vi "Day 8-2.vi"() -> ()   [LabVIEW 2019, in "Day 8.lvlib"]
uses:
  Day 8.lvlib
panel:
  out "Array 2":string[](array[string])=["4071", "6468", "3280", "8950", "2870", "3397", "3219", "7938", "9511", "6798", "2769", "3672", "6734", "0784", "4865", "7172", "1948", "3386", "6394", "6035", "6388", "4268", "5479", "3876", "9799", "2603", "7009", "2937", "8421", "2344", "6241", "3548", "9654", "4281", "2324", "3134", "1290", "2001", "6508", "3774", "2051", "8563", "6678", "9605", "9989", "6560", "5968", "0362", "3584", "8891", "4895", "8699", "2381", "9222", "1822", "5228", "1804", "0780", "9704", "9642", "2495", "4224", "0930", "3262", "3312", "9354", "9007", "1129", "1990", "5179", "8301", "5799", "8661", "6508", "4845", "6988", "8258", "9544", "0971", "3310", "8569", "1471", "9270", "1287", "7671", "0011", "0695", "1654", "2588", "9727", "1006", "9039", "2552", "5249", "3745", "3553", "3225", "8583", "4118", "3505", "6532", "5649", "3087", "8540", "7804", "6876", "7351", "1683", "8021", "2539", "2269", "0445", "7004", "5965", "3168", "3507", "5671", "3405", "6663", "3932", "1907", "1881", "6367", "0693", "1303", "7941", "1632", "0300", "4682", "0436", "9530", "0970", "2408", "0964", "3910", "9995", "1594", "0618", "7537", "2638", "4820", "6626", "2007", "8972", "4462", "0209", "4073", "9919", "4147", "2885", "6588", "3629", "1539", "0686", "7248", "1846", "0806", "9160", "6565", "9606", "5448", "1654", "8728", "7302", "9365", "5351", "1478", "9649", "3370", "6871", "0242", "3636", "4933", "6608", "5974", "7251", "2822", "5889", "2763", "9681", "2230", "1352", "2526", "3487", "4732", "5051", "0132", "6767", "1347", "2326", "2292", "0408", "2225", "6385", "0328", "2206", "5424", "2763", "3506", "8859"]
  out "Array":i32[](array[numeric])=[4071, 6468, 3280, 8950, 2870, 3397, 3219, 7938, 9511, 6798, 2769, 3672, 6734, 784, 4865, 7172, 1948, 3386, 6394, 6035, 6388, 4268, 5479, 3876, 9799, 2603, 7009, 2937, 8421, 2344, 6241, 3548, 9654, 4281, 2324, 3134, 1290, 2001, 6508, 3774, 2051, 8563, 6678, 9605, 9989, 6560, 5968, 362, 3584, 8891, 4895, 8699, 2381, 9222, 1822, 5228, 1804, 780, 9704, 9642, 2495, 4224, 930, 3262, 3312, 9354, 9007, 1129, 1990, 5179, 8301, 5799, 8661, 6508, 4845, 6988, 8258, 9544, 971, 3310, 8569, 1471, 9270, 1287, 7671, 11, 695, 1654, 2588, 9727, 1006, 9039, 2552, 5249, 3745, 3553, 3225, 8583, 4118, 3505, 6532, 5649, 3087, 8540, 7804, 6876, 7351, 1683, 8021, 2539, 2269, 445, 7004, 5965, 3168, 3507, 5671, 3405, 6663, 3932, 1907, 1881, 6367, 693, 1303, 7941, 1632, 300, 4682, 436, 9530, 970, 2408, 964, 3910, 9995, 1594, 618, 7537, 2638, 4820, 6626, 2007, 8972, 4462, 209, 4073, 9919, 4147, 2885, 6588, 3629, 1539, 686, 7248, 1846, 806, 9160, 6565, 9606, 5448, 1654, 8728, 7302, 9365, 5351, 1478, 9649, 3370, 6871, 242, 3636, 4933, 6608, 5974, 7251, 2822, 5889, 2763, 9681, 2230, 1352, 2526, 3487, 4732, 5051, 132, 6767, 1347, 2326, 2292, 408, 2225, 6385, 328, 2206, 5424, 2763, 3506, 8859]
  out "Resolt":i32=940724
  out "array":string[][](array[string])=[["ecgabfd gfbe dgbeaf aeg gfbda eg bgdcaf efgdca abced eadgb", " begf decgfa aeg eg"], ["ebfg bfgdea gaf gf baedgc dafec cfdabg ecfabgd fdgea dbaeg", " gaedbc egbf dbgcea dagfebc"], ["cfadeg ca bacg dfabe dgcbf dbegafc dac afbdgc gcbedf bfcda", " fbdac adbef bgcdfae dcagfe"], ["eag cdgfae cbdge ae fcgad eabdfg ecaf gefbadc dgafcb degca", " dacbefg fcdage agdcf fedagb"], ["dga edac gdfbea bgdfec da cfbga dbgec cadgb bdgace dcbfage", " acgfb gaecbfd dag gedfab"], ["cefb fb abcgefd fagbde fcbgae faecg cbadg cbfga bfa agcdef", " gbacf agbfc bgcaef baf"], ["ebdacf cbgfae cgdebaf afdcb gabdc df cdf eafd ecabf begdfc", " cbdaf gdabc fd cbefda"], ["ge daebc fcagb fdebac gaed ecabg egc gacedb cbdfeg adcfbeg", " gec gebdca ebagc adbgcfe"], ["bgfade gcefbd eafgd fcae cadgf gcf dgcba cfdega cagbdfe cf", " cdgeaf agfed cf cf"], ["abfge ebac acfegbd bc fcged gbfec cfgbad fecabg agbfde fcb", " aefgdb cfb egbfca cbfaedg"], ["dfcbag gda dcafe gcdeb ag ecgdaf edagc bcdaef gcbadfe gaef", " gbced dga cbadef fgecda"], ["cagb adgceb cdb cfgeda egfbd abcefd decag bc cgebd bgedfca", " cegbd dfegac dbc befdg"], ["cbfe bgefdc ceabdfg cf dbgaef gdfbac edcga gcfed dfc fbedg", " fgbaed fcd fcegd becf"], ["degabf bfg bcgaf gdacf dbfc gecfda gcaeb fagedbc adfgbc bf", " egbdfa gbf adfbceg dcfb"], ["dbfae dfbc ecadg cb cbdea fcebag fgadbec gadebf bec ceabfd", " dbfc bgfcead agbedf fdabe"], ["dafcge ecafbg cegaf egdac abegd cd debfca edc cgfd bfdeagc", " dec dc ecd dbgae"], ["fgabce bfa acbfegd fcegda bfgd acgfd bcaed bfcda bf cbagdf", " bf bafgcd bfdg dgbacfe"], ["fgea gad fcbgaed gdebc afdeb fagcbd cbfeda ag egfdba degab", " dgeab badge eacfbdg fdceba"], ["fabdce cagdb gcb bcefag degba dfagbc dgcf dcfab egfcabd cg", " befcda dbagc cbdgfa gcdf"], ["be fgaced fdeag badegf fdbea ebdg bea agfbec ebgadcf bcfad", " acdfge agbfce debaf dgafe"], ["cdfbeg bg fegca gdefac cadbf eadbcgf cgb egba gcfbea cagfb", " gfaced agfcb cbdfaeg cgfdabe"], ["fadcebg cgda ebfag adebc fcebdg fadbce gd begcda bdg gedba", " dcga fbage dcabef fcebadg"], ["bfcga adfbgc fbcdage gfedac ab gcfbe cgafd efabgd gab bdca", " gcafd cdba gba dfabgc"], ["bdfae gfa cdgabe egfba fg gfeadc acegb fgcb fbecgad ecafgb", " bgeaf agfecbd fga agdceb"], ["dgab ebfad cdefgb gbefd fab cefabg fegcbda aedcf ba ebadgf", " defbag afb gbfead dbefag"], ["cfabed ecabf cgafdeb bfc fecbgd dcab cb bfeda eagfc adfgeb", " fgcae dfbega ebcdfg fabec"], ["eb cbgaef eagcfbd caebd gaedbc badfc abe degac dgeb cgdeaf", " aeb gfaebc bceafg abcged"], ["gdecba ecbdgf def fcbade fd fdcg bgfae gdecb gfbde faegdbc", " fbage ecgdbf egdfb dfe"], ["dc dac egcadbf gadbe cgaebd abgcd geadbf agfced edcb gabfc", " agcbefd edbc bacfg cd"], ["gaebfc gdc cedbg dbeag cefd cd bcfgde cbgfda bcegf dabgecf", " bgdea dbgec fecd cfed"], ["afd dfcbga dcbeagf bfecda egbcdf dagec fa bgfa fdbcg fgadc", " egbcdf decga gbfa fa"], ["fg baefc gafeb dgaf cbgdea afegbd fbg cebgfd gaecdfb dbgae", " ebfag dgbae gafd abgedfc"], ["cbaed gedac cefgbda feba be cadebf gdcefb fcbad bde cdagbf", " bcadef cfgdab fdabc feab"], ["cfbdg fdgce adgcbf fb cbf acfegdb adgebc ebafdc dbacg agbf", " fgba fgced ecfdabg bf"], ["fceabd gfb agfdb deabg beacgf cfdgbae fcdg gf abfdc dfbgca", " dbaeg bfdga dgeab dfcg"], ["gfde facbde dcgbf fg gbf ecafgb cfgdbe ecdfb adcgb ecafbdg", " gcdbf fg cfbdg fdeg"], ["fbgdce bg bacefg decab cbg fecgd egdcfa dbfg egdcb fagdbce", " gb dcbea fedbgc fagecb"], ["abgcef fgbaedc dfaebg cgad ad egadcb abd cgbea bfecd cabde", " efbcd abdfeg afbegd ad"], ["fagecdb bcafg ecadfb fa bagecf cdgba efbdcg befgc fac agfe", " bdfcge ecgbf cfedba edagfcb"], ["dgf fcdbg cegbd fd bfcega daebgf dfca abgcf gafbdc fbeacgd", " bcfdg fdg dfg adcf"], ["deb cbdgae edfbac dbcgf fbecga gdfcbea bgdec ed ecabg egad", " bgcfd faedcb cageb ed"], ["gecfba dfagc afdbc adbcfg cag cabgdfe fdega cbdg dbacfe cg", " afcbdeg dabcf cbafed dcfga"], ["feab ae cbgfe agecf bgecda bgecdf eca gfebca fcdbgea cgfad", " bgdfec gcfbed eca cbdgaef"], ["fbaceg edcbaf dba becgd egafb degbfca fbadeg dafg da agebd", " fbdega gfebca acebdf gbefa"], ["dbce gfbec defgb ed efdagc def gfbeca abfgd bgfedc fcbgade", " fdbgce ebdfcg cgfbdea efcbgd"], ["abcdfg fcaegb egf dgcaf bdecf aged bdeacfg ge dgcafe gfcde", " acbgfd gcadf cgbdaf gafecb"], ["fb gbfaed eabgdc abcgef adcbfge dgfac fecb bgf fcbga cageb", " acebg cfeabg edgcab adgfbce"], ["fad ceafdg dcfag fbcadge geadbf deac da gcfea gdcfb efcagb", " aegdfb cgadf aefbcg bgdcf"], ["dagcbf ef dacfg gfdce egf ebdgc dfcgea fabdeg aefc ebdacfg", " gdefc dcfag bgdceaf acef"], ["dbegf eabcgd ebdafg fbdac cbg cefg eagbdfc cdbgf gdfbce cg", " eabcdgf gecadbf decgbf gc"], ["degf cbefd bfcdeg bfdaec bcage cfgdba fg fcg fbcge cefgdba", " fged cfgedab fdgceb efcbd"], ["cgbdae dbeca bcfdeg fcaged edgca be cbdaf ebd gfbadec egba", " cefdgab cdfega bcgeda agcbde"], ["cdfgea gbedacf gacbf cdb decag db edcabf gabedc dgeb bgdca", " bcfag bcgad ecdgfab bd"], ["ebcg cfgbae acgdbef eag agdfc ge edgabf cgefa facbe dacebf", " cbgefa agcfd fgcad dfgac"], ["beagcf dafcgbe da acd bedcf begacd cdbae cefadg bagd bgcae", " da fgbecad bdcef bfdec"], ["dg acgfebd fagecb bgeadf ebfgc gdb cdbgf dbafc gecd debfgc", " egcbf cafbd facbd afbegcd"], ["geabd cadefb ec eadgfcb cedag gdbeca dec gfbdae dcfag cbeg", " ec bdeafgc cbdafe ebcg"], ["be bfade caefgb eab gdbafe bedg agfdb edacfbg gdcabf daefc", " acfegb bae fecadgb bgcfea"], ["be acdfb cgfae cbe agbe fgeacbd adegcf bcfae bgcefa fgbecd", " cfabeg ecb efcdbg ageb"], ["afbg cfedb dacfgb fgdcb bgfedac cbdage bg acgdf fadceg dgb", " cdbgfa fgeadc bafg dfbce"], ["debfc efb adgbce ef fbadec dfcbg feac dacgebf aebdc eadgfb", " fcdgb efca cbdeaf edbca"], ["gcbde dgcbf dfc bfcgda df ceadgbf gcabf dbaf gcefab dfcega", " adfb egcdb dgbce bdfa"], ["egbdca bgfed baefd cfdgaeb gdefc gcbfed gcfead bg cfgb egb", " dcbage cbdgef dgfbe aedbcg"], ["dceaf fc fcge bgdaec agced dfbea cgeabdf adcfbg fdc egcfad", " fedca fadeb dabegc aedfb"], ["acfbgd efcda cfagd decg de efcgdab eabfc gdaecf dae bedfag", " fceda acdef ed cfeba"], ["defbcg ge egb eagbdc afdgcb cgbae fcadebg geda dcagb efcba", " gdecba abgce gbadc daeg"], ["afbd fadgce gbfdea fcgedb bf bgf gefda bfedgac bgcea gaebf", " bgfaed fdgecb fbgedc bfg"], ["cbafgd cbdge bc cbd bcef fgbde afgbde fgcbed dgebfca edcga", " cb cb acged fdgbec"], ["acgd dceagf dc bafde fbaceg ced cdfbge fdeca egcabfd cgefa", " dc egdcfa afegcd efcgbd"], ["bgdfac fb aebgc bfde bdecaf bfa aebcf edabfcg cgdeaf daefc", " decfa fb baf fcbdea"], ["bdfegc gebda gecbfa fedbg fed dgfc fabdec dbcagef fd gfcbe", " edcfbag dgfeb cdeafb fd"], ["gbeadf fdcga ecadb bceg ge egd dgebacf beafcd aedgc cgbade", " dabec dge begdac dgaebc"], ["begc dcgbfa eb dfeag eafgb bae bcgaf gfaebc fbagecd becfad", " gabdcfe fdcagb bgcdaf be"], ["eca febdcg fedag ecdaf fcba beagdc fcdeb ca dbefca acebfdg", " ebdcgf fdceb gecdab cedfbga"], ["decfbga abgdce gefd afd aecdbf gcfeda acgde cafbg fd fadcg", " edgf dafbceg egfd cedga"], ["faedgbc fbgaec dacb eba geacdb bcgefd ba bdegc eadbg gdaef", " dfcbge deabcg bfecadg gfcbaed"], ["egfacbd acdgf gecdab ebacf abcfed eg begf caegf aeg bfgeca", " dafbcge cadfg fbace cefdbag"], ["dgcfbae ac gbfeca badce gcad dfgcbe defab cea acgdbe dbgce", " cgdeba egcdb gcad cagd"], ["dcfg agdfbc caedfgb df bagecf daf gcafb ebcad fdbac agebdf", " bdfage fgdbac daf fd"], ["agefbd agcbfde egafb eg adge fge bfaced egdbcf daefb cabgf", " bagef afgbe eg efbcdg"], ["adfegb caefgb ade ecgd cafed dbfeacg de fgcae fbcda fgadce", " dbefgac eafcg gbaefc fedgac"], ["dbafg ecfga gfbae bae egdbac geabfc gcedfab ebcf eb cagdef", " be cbfe bae be"], ["cfgadbe eca bcfadg ebdgac adgcb ebdca adbfe egcb cadfeg ec", " adebgc feabd cae cgdfea"], ["caefdg cdfagbe fadbc afd eacbd fd bcadeg cgfba dacfeb bfed", " df afcgb fceabdg fda"], ["edcgaf cfbdag cbfdaeg ec cae bgeafc cdafe abfde decg gdcaf", " eca dbcafg aec ce"], ["fbgae cagef egdbac cg gcdafbe cfbg bgefda gce ceadf gebfac", " gadbce cdegba gc cg"], ["bafgecd bdf ecabfg dgbfe dcefg gbefa bdea bdfcga bd bgfdae", " cdfagb cfeabg faebgd fagbe"], ["afg dfcg fg eacdbg fgadeb cfdgea ecagd fcagebd eacfg bacfe", " fg dagecb egdca cfdg"], ["dac dc fgcd agbecf gcdaef agbed edcabf fgace caged faecdbg", " dabge gceaf gdafecb cdafgeb"], ["aefbg egf bagcf afegdc dfgceab begd gafebd eafbd eg fabcde", " egadfb feg bgcfa efg"], ["fa debfg acgfdb eagbc dcebagf cedfbg dafe baf febga eagbfd", " af cbfdga dcfgab befcdg"], ["db dbfe fdbga cafdg adgceb egbfa dbg bgfdcea ceagbf befagd", " afdbge dceabg gdfab fdaegb"], ["fgeacdb cadg dfg edfga fdagce dg dfaec gebfa cbefgd defabc", " geabf dfaec cfdae faegb"], ["abdce bafcg gdecaf cegba fbcadge adbcfe degb eg bdcgae eag", " abdec facbg edgb ebagcd"], ["bcaef fg dgbcae adegb bafeg feadcgb egbfad fdgb fecagd efg", " agfeb fge fdgb eadgb"], ["dbfage cdab bgcaef ecb cb dgfce dfbce fedbgac deabf beadcf", " cbfed dabfe ebadf cefbd"], ["gcedb ceafdg dcg gecdfb dcfaeb cg egdba befdgac fdceb gcfb", " begdc bedag eadgb dfecb"], ["bf dbcgea eabdfc feb gbfeac fagb becga fcdaebg dcgef gecfb", " efbdcag abceg gcdabef gcbef"], ["ged dagfbe eg cgfe bgfacde gedac dceba agcfd cadegf gcfdba", " gefc ge ge acegfbd"], ["gfabed aecdgf ecbag dge gbdae befd bfgad fdcabeg de fagbdc", " egbad afdbg dgacef gdafb"], ["dabfegc gbcad gafd acd da fgbadc ecdabf bfgca fcabge gbdec", " gbface fgcab bdgac ebdcg"], ["afbceg cdgfb gb afcbed dfcbge gbf adfgc fecbgad egdb bcdfe", " fedbc cfeabd edbg cfebgd"], ["cbdae gc gdfc ebgdf gcafbe fbaecdg gbedc ecg fbgecd fdebag", " gcedb ebgafc acfgdeb ceg"], ["bdce efacgd dgfbc ebfgad bcfga gdc fgbedac egdfb dc bfdgce", " bagdfec efdgb ecbd fdaegc"], ["bdgefc fbca bc gfbcae fdcgae gdaeb cbega gcb efagdcb feagc", " gcb bacefgd ecdbgf cfab"], ["fdbe defcbga adf cfgeba gcdae bacef cfadgb df fdeca dcefba", " cbegfa degfcab fad acgfbe"], ["gabfdc ebcfd bacgf da fcgbea aedbfcg gdfa eadcbg cdfba abd", " dab dabcf afcgb ad"], ["gb bfgcae dbgf cadeg bagdc gefadcb gbc acdbef cgabdf dbafc", " gb fbdcae afdbgce dabgc"], ["cfgadbe agecfd ea gedfc edafc fage fbdgce ead aecdbg fabdc", " fcbdage cdbage fbadc ae"], ["decgbaf edcgba afgd aebgfd da bfeag gfbcae bad cebfd bfeda", " ecfdb eagbf efdba eabgdf"], ["cfdbae dc gbdef fbedag egbfcd gafec edc edacgbf egdcf bdgc", " fceag gacfe daegfb bgdcef"], ["cbgda egdfb agebd cgedfb aed bfgdcea ae agdefb efab facedg", " gdcaef aefb faeb begfd"], ["fdc begdf adecg gfaced cf efac abedfgc cbedag gdbacf fecgd", " cdf fbgadc cabgdf acfe"], ["fedbg gabfe feda gde fcdbg de dbegacf bdfaeg abcdeg cegbfa", " bgaef gadebf efgbac gbefa"], ["dgf fgdbea dg dafcb gdec edcfbga dbegfc gbdcf cfbge gcebfa", " bdfgc dg egcfab bcdafge"], ["ceg daecb gcfdea fgacbe ecadbfg eg gbacdf cgabf ebfg ecabg", " acgeb bfgca geacdf cge"], ["ge geabf gea abecgf fdabg caedbf egbc cgebafd cbfea agdefc", " feabc bcdafe age eg"], ["gecdba ebdfg gcdef ecf cefadb fgac cf ecgafd cbfgead adgec", " dfecg afcg bcfead ecadg"], ["gd cbfad fdagb cfbeag fabge efabdg aged bdgfec dgf gbfadec", " acefgb eabfgc becagf bfgda"], ["ebgc fedabcg fdbgce fdebg eg badgf ebcdf edg adcfeb cfgade", " bgefd cbgefd bgefd abfdg"], ["dgbfc abecfg gcdab fcgdbe dfge cbdfea defbc fgc dabgefc gf", " gf dbgecf bafgec cgf"], ["degbac fda cdbag eafgbcd df fdbc agfdcb dabfg fbgea fcgade", " fd bdceafg fdagbce df"], ["cedaf fgeabc egdbf gbaedcf aeg cgda dfaeg cfdbea fagdce ga", " febadc gefad bfacde gae"], ["gea ebfgdc bcae cgafd abecfgd gbced ea gbdeaf dcgae gebcda", " efgdab fcegdb cbgade acged"], ["cdabgef gb fceag fgb bfdgac gbcfa cbadfe dfcegb fbdca bgda", " bg cbgfa dcfgeb afcgb"], ["fcbage adefc gceda bdegca cbeag dgeb efacdgb cfbgda adg dg", " gad gabced gebd dg"], ["ecbdga gedbf dafeg faecbdg eacfg dbaf ad dbfcge gda dfbeag", " ad gfbcde dgfea aecfg"], ["agfbde begfca bca baegc bc bcef ecdgbfa adegc bgaef acbfdg", " fdbcag baecg cgdbaf bcdagf"], ["beafc badfc daecfb fd fad fdec badefg cbdag fbecgad gecfab", " dcfe cbgeaf gdcfabe agdbc"], ["caedgbf fcgead ca gbadf abcd adcfbg fegbc dfaebg gfbac agc", " fcgeda dbac afcgb dafebg"], ["gdfeb gdbafe bc ecb ebfagdc bgfce gfeca fdcbge aebdcf bcdg", " cdfbeg gdbfe gefcb dbcafe"], ["gfbca gcdfe dbafgc cafgbe eacfbgd cdb agdb db cgdbf ecdbaf", " adfcbe abdgfc cdb fcabed"], ["bcdaf fbed edbac cdaegf ed dbgaecf edc ebgac dbagfc fdbace", " cbgae efdb gcdafe gbafedc"], ["cdfba cbdfae cfga bafdgc aedfgbc dbgef dag adgfb bdaegc ag", " ebacgd adfgcb bdaefc gfac"], ["caefd ce abfdc egcbdf cfe fgaced bdgfea gcae fadcbge eagfd", " fcdae fgecad ec cbefgd"], ["eafbd deb aefdg bd aecfbg bdcf abcfe gebcdaf agdbec bcaedf", " dbcfae abfecd efabcd cbafe"], ["bdafeg efg gfcdae bagfd dfacgb ef dgfecba befa efbdg dbceg", " fe gadbf aebfdg afeb"], ["cgbef ceb bfdgcae gedbac acgfbe be gceafd eacfg fcdgb fbea", " abcedg dcgefa be fcegadb"], ["gacb gfbaedc fagdc baf gadcef bfcdea fgebd gfabd cfdgba ba", " baf cadfg gbfad fab"], ["gafce df cbdfge gfd gdecb gecdf fdeb cadbeg agdbcf abgdcef", " cgfea abgcde decgf fgcdbea"], ["egdbf cbfgde aed befa gfdbae ea abcgd edfcga bcaegdf agdbe", " bfae cagbfde cbgda gedcaf"], ["eb dfbacge dbgae becafg abe gadfb cdega cedagb ecfgad debc", " cfgeda fagedc afdbg fdcega"], ["efcba becagd gafcdbe eafdbg dagbcf agfbd gefd de bfaed deb", " fabce bgaedc ceadbg bed"], ["cbaedf fdgebca gdbe dabce eag ge bacge bagcf decfga bgecda", " defgabc bceagd aeg gbacf"], ["dgeabf aefgcdb ad bcfae bdacf dacg bgfdc ebfdgc gfdbac abd", " dcga adgc decfbg bafce"], ["fgcba cbdfeag dagfb dcgbaf dcaegb ecbafg bdg bd fcbd faegd", " bgdaec feadg cbdage dcgafb"], ["bdc dcfgeb ebgca bdea bdcga abfecg gdcaf bd aecdbfg aebgdc", " bade bdecgf bdc cbadg"], ["bcdaeg facgbd caedfb aefdb dgfbe eba ae dcegfab fcea fbcad", " cbafed baecdf ae ceabfd"], ["efcbg egd dg cabgef bfdceag fgcbde fdcea gdfb dgebca dfcge", " fdgb gd fbgd deg"], ["cbgdfa ebgcfa abdge bdeca efcgbad cd fbedac abecf adc edcf", " agebd gfabedc dabfegc abfce"], ["edg abdgce gcefb dcbge dgabfe gcdab de cdebfga cdae fdabcg", " gbdafc agcdb dgfceab bafgdec"], ["acdb dgbfec eagfcdb dafbec cae ebdfc ca gfaed acdef gfebac", " defac begdfc daegf fdeacb"], ["cgedf gfadce debgcf fedagcb aefbc bcdagf db ebfcd bfd begd", " db cgfde dbefc gedcfb"], ["afcbegd dcfge edgbf bdg fabd dabfeg gaebdc abgecf gfeab db", " debacg gfbaec fadbegc afcgbe"], ["fcbg cdegf ecdga eacdfb befdg dcf fc dfegba dbfgce agdfcbe", " dcf adcge fbcg dgaefbc"], ["bcfea fcbead ecd cgeafb aebcgd bfed bcgedfa de cadfg fedac", " de egadfbc debf bfagec"], ["efcdabg afecbd defba cabfd ebca cgdaf dfabeg bc efcdbg fbc", " bgdefc afcgebd gdefcb efabgd"], ["edbaf agfbcde gbfcae ag dega aefcdb dfbega dfgbc afdgb bag", " dagefb ga decbfa aecbgf"], ["cbdg aegbcfd badce dgaebf abdcfe gad cgeda gd fcage ceagbd", " fdcaeb dbeca beafdc bdace"], ["decb dagfe dcgbafe fecbda acfdb adfbcg agefbc fec ec faced", " fcadeb cdagfb agbfce gcfdba"], ["acdbef dgca gbfae agecfdb ebdcg bda bgeda gedbfc ad bcadge", " cgdbe cdag dcga efdcgab"], ["gc efbdg eadcf ebcafg adecgf gfdbaec gcf gcda dcgfe dcbaef", " gc acedbf fcead gdca"], ["bfgce dabfg ecdf cebgfa dfegb ed deb fecbgda becgda cfbedg", " cdgbefa ebd gafdb cdgefba"], ["ce gecb ecd debaf ecdfb dcfega dagcbef fbgcd bdcgaf dcgfeb", " dec dfbec agcfed bedfa"], ["cgbfd gb dcafg gadb gbfcea bcfdeag fcbde fbg gcbfad agdfec", " dcfgab bfgdc dfaceg dfgac"], ["bgacef cdagf bgdcae gd dag dbagfc fecagbd fdbg cfead agbfc", " gfcba adgcf facgb gd"], ["efdc adbgc gec acfgde feadg gbecaf fbdgae agdec daefbgc ce", " ec cedf cge bdfagce"], ["aecdbg cabfe acfgeb bcefda fgac fdgeb afdcbge bcg cebfg gc", " gcbfae febcda facg baefcg"], ["dgbafce gfacdb gecb dcaefg gfaeb egf gebacf bdefa bgcaf eg", " abfge fgabe fge deagfc"], ["ceafdb dcbega afd gdbeaf fdgea fgeac gbade cbfadeg fd dfbg", " adbcge gdcfeab afd fd"], ["dacegf ed dfcbg cfgea dcfge fcgdbae acgbef ced eagd abefcd", " dfbeac fgcdb geda dbfgc"], ["egbcdf ecbdga afegc aefdbgc dgeca dge dg dcfbae dgab cdbea", " gcead eabdcf gdeac cfadbe"], ["gca fceagd fdgbc ga fecab fgcabed bgcaf cdbfge adbg acdfgb", " agdb bfadcg bfgac gbfca"], ["acgdeb baefd fa gdfa bgdea bdcfe fdagebc fdgbea ecfgba fab", " adbecg agcbed febagc feagcdb"], ["fedagc dcfge ef bgdcf gdceba egf fead edcag gfbaec fdgaebc", " cgade aecfdg efg eadf"], ["dbagf gcdefab fc badfc cbaed gfadbe dgfc gfbcad gaebfc bcf", " cfb cdbea bdagf fc"], ["bae be gcadeb dbge dgebacf eagcd geabc fbcga eagfdc edbafc", " gcabf ecdfbag afbcg cbgfa"], ["bd gdbcf cbfegd cfbeag febdagc fbd fcgeb decb afgbed dfgac", " cbefg eadcbfg cbegfad egdfcb"], ["febacg dega cegfd cefda ae agebcfd abcdf eca defacg ecgfbd", " badcf cae bdcefg acedf"], ["geabcd gdbcfa gaedc cbeagf bdgeacf gdefc bdacg ae adbe cae", " gcebad agfbdc gefbcad ea"], ["fa bfdacge adecgb eacf bdfgac gfdbe aegdc egacfd gadfe fga", " gedfb egfbd efagd dagfbc"], ["gcdb dg beagdf feacg cebgdfa afbcd adcgf dbfcga ebfdac agd", " gd acdfg dcbaf gacfe"], ["aefgbd cgfdb gfdea eabfgc dcgfe cfe ceda gdcaef ce fdeabgc", " bdcgf edgaf cbdfg egfbda"], ["facegb cfdabeg bd cedgbf adcfeb cfabe cdb eadb cgdfa dfbca", " dfbca eadb adecbgf bdc"], ["bacfeg agfcdeb acegf gfcade ecagbd fdbag afegd cdfe ed edg", " dfce egd degaf dagfb"], ["df gdfcea efbadg cegafbd eacfd fad cedbga dgaec dfcg fbcea", " caedg dgafbe edgac df"], ["bfdac cdbgfa cefbgd bfag afgbdec cdgafe cbfdg acf ecbda fa", " dgcfae af cabfd beadc"], ["befgd dea ecab baefcd gfbcad ea bafcd dbcgefa afebd cadfeg", " gfbadc eda cadgfb eda"], ["gf cgadb gebf becfdga gaefcd febac gcbaf cbfdea bfgeac fag", " fg afcbg efbg afg"], ["ba aebg gafdceb bca bdacg dagcf fcbdae gcbed cadebg bgcefd", " dcagf gdabc afgcd edcfgb"], ["de dbec bfaecdg gdfeca fegcb edg dbgaf fceabg febcgd bgdef", " afdbg adbfg debfgc bdgfa"], ["afbced adebfg efagdbc caebf afgec ecgb ega eg fgdac acegfb", " aedgbf cbge egbfda badfgec"], ["fg gbfcdea eafbcd fdaeb cdage egf agdefb fdcbge efgda fgab", " deacg cdage gedca adfeb"], ["gde gbdc dg fdgec dfaegb fedca bcgefd fbeacg gadecbf fcbeg", " cgfabe edcgf fgeabdc cbefg"], ["befcdg agbcef fcbdeag gdfae bdecf eab fcdeab ab efbad bcad", " cfgeba befda aefgd degbcfa"], ["abcef dbfaegc aefcg dcgbae fbcg efgacb cg cdabfe gec dfeag", " dgfae gdefa agcbde afbced"], ["dgf fcbega afdbeg fgabe dg efadg bged adfbceg agbcfd fedca", " aefgb begd fceda debg"], ["cdgaeb ba befgdca defbc gdecaf bae gabc afgdeb gedac decab", " fbecd bae gdecfa edcba"], ["ebagfd dfg dcbaeg dgbceaf gf gacdf fcade gacbd gcfb fbagcd", " adgfc acbgd edbagf degabc"], ["gba eagbcf gb gbacf dacgebf bceg gcafed acfeg acbfd adegfb", " abfcdeg dbcfage faecg afebgc"]]
  in  "String":string="ecgabfd gfbe dgbeaf aeg gfbda eg bgdcaf efgdca abced eadgb | begf decgfa aeg eg\nebfg bfgdea gaf gf baedgc dafec cfdabg ecfabgd fdgea dbaeg | gaedbc egbf dbgcea dagfebc\ncfadeg ca bacg dfabe dgcbf dbegafc dac afbdgc gcbedf bfcda | fbdac adbef bgcdfae dcagfe\neag cdgfae cbdge ae fcgad eabdfg ecaf gefbadc dgafcb degca | dacbefg fcdage agdcf fedagb\ndga edac gdfbea bgdfec da cfbga dbgec cadgb bdgace dcbfage | acgfb gaecbfd dag gedfab\ncefb fb abcgefd fagbde fcbgae faecg cbadg cbfga bfa agcdef | gbacf agbfc bgcaef baf\nebdacf cbgfae cgdebaf afdcb gabdc df cdf eafd ecabf begdfc | cbdaf gdabc fd cbefda\nge daebc fcagb fdebac gaed ecabg egc gacedb cbdfeg adcfbeg | gec gebdca ebagc adbgcfe\nbgfade gcefbd eafgd fcae cadgf gcf dgcba cfdega cagbdfe cf | cdgeaf agfed cf cf\nabfge ebac acfegbd bc fcged gbfec cfgbad fecabg agbfde fcb | aefgdb cfb egbfca cbfaedg\ndfcbag gda dcafe gcdeb ag ecgdaf edagc bcdaef gcbadfe gaef | gbced dga cbadef fgecda\ncagb adgceb cdb cfgeda egfbd abcefd decag bc cgebd bgedfca | cegbd dfegac dbc befdg\ncbfe bgefdc ceabdfg cf dbgaef gdfbac edcga gcfed dfc fbedg | fgbaed fcd fcegd becf\ndegabf bfg bcgaf gdacf dbfc gecfda gcaeb fagedbc adfgbc bf | egbdfa gbf adfbceg dcfb\ndbfae dfbc ecadg cb cbdea fcebag fgadbec gadebf bec ceabfd | dbfc bgfcead agbedf fdabe\ndafcge ecafbg cegaf egdac abegd cd debfca edc cgfd bfdeagc | dec dc ecd dbgae\nfgabce bfa acbfegd fcegda bfgd acgfd bcaed bfcda bf cbagdf | bf bafgcd bfdg dgbacfe\nfgea gad fcbgaed gdebc afdeb fagcbd cbfeda ag egfdba degab | dgeab badge eacfbdg fdceba\nfabdce cagdb gcb bcefag degba dfagbc dgcf dcfab egfcabd cg | befcda dbagc cbdgfa gcdf\nbe fgaced fdeag badegf fdbea ebdg bea agfbec ebgadcf bcfad | acdfge agbfce debaf dgafe\ncdfbeg bg fegca gdefac cadbf eadbcgf cgb egba gcfbea cagfb | gfaced agfcb cbdfaeg cgfdabe\nfadcebg cgda ebfag adebc fcebdg fadbce gd begcda bdg gedba | dcga fbage dcabef fcebadg\nbfcga adfbgc fbcdage gfedac ab gcfbe cgafd efabgd gab bdca | gcafd cdba gba dfabgc\nbdfae gfa cdgabe egfba fg gfeadc acegb fgcb fbecgad ecafgb | bgeaf agfecbd fga agdceb\ndgab ebfad cdefgb gbefd fab cefabg fegcbda aedcf ba ebadgf | defbag afb gbfead dbefag\ncfabed ecabf cgafdeb bfc fecbgd dcab cb bfeda eagfc adfgeb | fgcae dfbega ebcdfg fabec\neb cbgaef eagcfbd caebd gaedbc badfc abe degac dgeb cgdeaf | aeb gfaebc bceafg abcged\ngdecba ecbdgf def fcbade fd fdcg bgfae gdecb gfbde faegdbc | fbage ecgdbf egdfb dfe\ndc dac egcadbf gadbe cgaebd abgcd geadbf agfced edcb gabfc | agcbefd edbc bacfg cd\ngaebfc gdc cedbg dbeag cefd cd bcfgde cbgfda bcegf dabgecf | bgdea dbgec fecd cfed\nafd dfcbga dcbeagf bfecda egbcdf dagec fa bgfa fdbcg fgadc | egbcdf decga gbfa fa\nfg baefc gafeb dgaf cbgdea afegbd fbg cebgfd gaecdfb dbgae | ebfag dgbae gafd abgedfc\ncbaed gedac cefgbda feba be cadebf gdcefb fcbad bde cdagbf | bcadef cfgdab fdabc feab\ncfbdg fdgce adgcbf fb cbf acfegdb adgebc ebafdc dbacg agbf | fgba fgced ecfdabg bf\nfceabd gfb agfdb deabg beacgf cfdgbae fcdg gf abfdc dfbgca | dbaeg bfdga dgeab dfcg\ngfde facbde dcgbf fg gbf ecafgb cfgdbe ecdfb adcgb ecafbdg | gcdbf fg cfbdg fdeg\nfbgdce bg bacefg decab cbg fecgd egdcfa dbfg egdcb fagdbce | gb dcbea fedbgc fagecb\nabgcef fgbaedc dfaebg cgad ad egadcb abd cgbea bfecd cabde | efbcd abdfeg afbegd ad\nfagecdb bcafg ecadfb fa bagecf cdgba efbdcg befgc fac agfe | bdfcge ecgbf cfedba edagfcb\ndgf fcdbg cegbd fd bfcega daebgf dfca abgcf gafbdc fbeacgd | bcfdg fdg dfg adcf\ndeb cbdgae edfbac dbcgf fbecga gdfcbea bgdec ed ecabg egad | bgcfd faedcb cageb ed\ngecfba dfagc afdbc adbcfg cag cabgdfe fdega cbdg dbacfe cg | afcbdeg dabcf cbafed dcfga\nfeab ae cbgfe agecf bgecda bgecdf eca gfebca fcdbgea cgfad | bgdfec gcfbed eca cbdgaef\nfbaceg edcbaf dba becgd egafb degbfca fbadeg dafg da agebd | fbdega gfebca acebdf gbefa\ndbce gfbec defgb ed efdagc def gfbeca abfgd bgfedc fcbgade | fdbgce ebdfcg cgfbdea efcbgd\nabcdfg fcaegb egf dgcaf bdecf aged bdeacfg ge dgcafe gfcde | acbgfd gcadf cgbdaf gafecb\nfb gbfaed eabgdc abcgef adcbfge dgfac fecb bgf fcbga cageb | acebg cfeabg edgcab adgfbce\nfad ceafdg dcfag fbcadge geadbf deac da gcfea gdcfb efcagb | aegdfb cgadf aefbcg bgdcf\ndagcbf ef dacfg gfdce egf ebdgc dfcgea fabdeg aefc ebdacfg | gdefc dcfag bgdceaf acef\ndbegf eabcgd ebdafg fbdac cbg cefg eagbdfc cdbgf gdfbce cg | eabcdgf gecadbf decgbf gc\ndegf cbefd bfcdeg bfdaec bcage cfgdba fg fcg fbcge cefgdba | fged cfgedab fdgceb efcbd\ncgbdae dbeca bcfdeg fcaged edgca be cbdaf ebd gfbadec egba | cefdgab cdfega bcgeda agcbde\ncdfgea gbedacf gacbf cdb decag db edcabf gabedc dgeb bgdca | bcfag bcgad ecdgfab bd\nebcg cfgbae acgdbef eag agdfc ge edgabf cgefa facbe dacebf | cbgefa agcfd fgcad dfgac\nbeagcf dafcgbe da acd bedcf begacd cdbae cefadg bagd bgcae | da fgbecad bdcef bfdec\ndg acgfebd fagecb bgeadf ebfgc gdb cdbgf dbafc gecd debfgc | egcbf cafbd facbd afbegcd\ngeabd cadefb ec eadgfcb cedag gdbeca dec gfbdae dcfag cbeg | ec bdeafgc cbdafe ebcg\nbe bfade caefgb eab gdbafe bedg agfdb edacfbg gdcabf daefc | acfegb bae fecadgb bgcfea\nbe acdfb cgfae cbe agbe fgeacbd adegcf bcfae bgcefa fgbecd | cfabeg ecb efcdbg ageb\nafbg cfedb dacfgb fgdcb bgfedac cbdage bg acgdf fadceg dgb | cdbgfa fgeadc bafg dfbce\ndebfc efb adgbce ef fbadec dfcbg feac dacgebf aebdc eadgfb | fcdgb efca cbdeaf edbca\ngcbde dgcbf dfc bfcgda df ceadgbf gcabf dbaf gcefab dfcega | adfb egcdb dgbce bdfa\negbdca bgfed baefd cfdgaeb gdefc gcbfed gcfead bg cfgb egb | dcbage cbdgef dgfbe aedbcg\ndceaf fc fcge bgdaec agced dfbea cgeabdf adcfbg fdc egcfad | fedca fadeb dabegc aedfb\nacfbgd efcda cfagd decg de efcgdab eabfc gdaecf dae bedfag | fceda acdef ed cfeba\ndefbcg ge egb eagbdc afdgcb cgbae fcadebg geda dcagb efcba | gdecba abgce gbadc daeg\nafbd fadgce gbfdea fcgedb bf bgf gefda bfedgac bgcea gaebf | bgfaed fdgecb fbgedc bfg\ncbafgd cbdge bc cbd bcef fgbde afgbde fgcbed dgebfca edcga | cb cb acged fdgbec\nacgd dceagf dc bafde fbaceg ced cdfbge fdeca egcabfd cgefa | dc egdcfa afegcd efcgbd\nbgdfac fb aebgc bfde bdecaf bfa aebcf edabfcg cgdeaf daefc | decfa fb baf fcbdea\nbdfegc gebda gecbfa fedbg fed dgfc fabdec dbcagef fd gfcbe | edcfbag dgfeb cdeafb fd\ngbeadf fdcga ecadb bceg ge egd dgebacf beafcd aedgc cgbade | dabec dge begdac dgaebc\nbegc dcgbfa eb dfeag eafgb bae bcgaf gfaebc fbagecd becfad | gabdcfe fdcagb bgcdaf be\neca febdcg fedag ecdaf fcba beagdc fcdeb ca dbefca acebfdg | ebdcgf fdceb gecdab cedfbga\ndecfbga abgdce gefd afd aecdbf gcfeda acgde cafbg fd fadcg | edgf dafbceg egfd cedga\nfaedgbc fbgaec dacb eba geacdb bcgefd ba bdegc eadbg gdaef | dfcbge deabcg bfecadg gfcbaed\negfacbd acdgf gecdab ebacf abcfed eg begf caegf aeg bfgeca | dafbcge cadfg fbace cefdbag\ndgcfbae ac gbfeca badce gcad dfgcbe defab cea acgdbe dbgce | cgdeba egcdb gcad cagd\ndcfg agdfbc caedfgb df bagecf daf gcafb ebcad fdbac agebdf | bdfage fgdbac daf fd\nagefbd agcbfde egafb eg adge fge bfaced egdbcf daefb cabgf | bagef afgbe eg efbcdg\nadfegb caefgb ade ecgd cafed dbfeacg de fgcae fbcda fgadce | dbefgac eafcg gbaefc fedgac\ndbafg ecfga gfbae bae egdbac geabfc gcedfab ebcf eb cagdef | be cbfe bae be\ncfgadbe eca bcfadg ebdgac adgcb ebdca adbfe egcb cadfeg ec | adebgc feabd cae cgdfea\ncaefdg cdfagbe fadbc afd eacbd fd bcadeg cgfba dacfeb bfed | df afcgb fceabdg fda\nedcgaf cfbdag cbfdaeg ec cae bgeafc cdafe abfde decg gdcaf | eca dbcafg aec ce\nfbgae cagef egdbac cg gcdafbe cfbg bgefda gce ceadf gebfac | gadbce cdegba gc cg\nbafgecd bdf ecabfg dgbfe dcefg gbefa bdea bdfcga bd bgfdae | cdfagb cfeabg faebgd fagbe\nafg dfcg fg eacdbg fgadeb cfdgea ecagd fcagebd eacfg bacfe | fg dagecb egdca cfdg\ndac dc fgcd agbecf gcdaef agbed edcabf fgace caged faecdbg | dabge gceaf gdafecb cdafgeb\naefbg egf bagcf afegdc dfgceab begd gafebd eafbd eg fabcde | egadfb feg bgcfa efg\nfa debfg acgfdb eagbc dcebagf cedfbg dafe baf febga eagbfd | af cbfdga dcfgab befcdg\ndb dbfe fdbga cafdg adgceb egbfa dbg bgfdcea ceagbf befagd | afdbge dceabg gdfab fdaegb\nfgeacdb cadg dfg edfga fdagce dg dfaec gebfa cbefgd defabc | geabf dfaec cfdae faegb\nabdce bafcg gdecaf cegba fbcadge adbcfe degb eg bdcgae eag | abdec facbg edgb ebagcd\nbcaef fg dgbcae adegb bafeg feadcgb egbfad fdgb fecagd efg | agfeb fge fdgb eadgb\ndbfage cdab bgcaef ecb cb dgfce dfbce fedbgac deabf beadcf | cbfed dabfe ebadf cefbd\ngcedb ceafdg dcg gecdfb dcfaeb cg egdba befdgac fdceb gcfb | begdc bedag eadgb dfecb\nbf dbcgea eabdfc feb gbfeac fagb becga fcdaebg dcgef gecfb | efbdcag abceg gcdabef gcbef\nged dagfbe eg cgfe bgfacde gedac dceba agcfd cadegf gcfdba | gefc ge ge acegfbd\ngfabed aecdgf ecbag dge gbdae befd bfgad fdcabeg de fagbdc | egbad afdbg dgacef gdafb\ndabfegc gbcad gafd acd da fgbadc ecdabf bfgca fcabge gbdec | gbface fgcab bdgac ebdcg\nafbceg cdgfb gb afcbed dfcbge gbf adfgc fecbgad egdb bcdfe | fedbc cfeabd edbg cfebgd\ncbdae gc gdfc ebgdf gcafbe fbaecdg gbedc ecg fbgecd fdebag | gcedb ebgafc acfgdeb ceg\nbdce efacgd dgfbc ebfgad bcfga gdc fgbedac egdfb dc bfdgce | bagdfec efdgb ecbd fdaegc\nbdgefc fbca bc gfbcae fdcgae gdaeb cbega gcb efagdcb feagc | gcb bacefgd ecdbgf cfab\nfdbe defcbga adf cfgeba gcdae bacef cfadgb df fdeca dcefba | cbegfa degfcab fad acgfbe\ngabfdc ebcfd bacgf da fcgbea aedbfcg gdfa eadcbg cdfba abd | dab dabcf afcgb ad\ngb bfgcae dbgf cadeg bagdc gefadcb gbc acdbef cgabdf dbafc | gb fbdcae afdbgce dabgc\ncfgadbe agecfd ea gedfc edafc fage fbdgce ead aecdbg fabdc | fcbdage cdbage fbadc ae\ndecgbaf edcgba afgd aebgfd da bfeag gfbcae bad cebfd bfeda | ecfdb eagbf efdba eabgdf\ncfdbae dc gbdef fbedag egbfcd gafec edc edacgbf egdcf bdgc | fceag gacfe daegfb bgdcef\ncbgda egdfb agebd cgedfb aed bfgdcea ae agdefb efab facedg | gdcaef aefb faeb begfd\nfdc begdf adecg gfaced cf efac abedfgc cbedag gdbacf fecgd | cdf fbgadc cabgdf acfe\nfedbg gabfe feda gde fcdbg de dbegacf bdfaeg abcdeg cegbfa | bgaef gadebf efgbac gbefa\ndgf fgdbea dg dafcb gdec edcfbga dbegfc gbdcf cfbge gcebfa | bdfgc dg egcfab bcdafge\nceg daecb gcfdea fgacbe ecadbfg eg gbacdf cgabf ebfg ecabg | acgeb bfgca geacdf cge\nge geabf gea abecgf fdabg caedbf egbc cgebafd cbfea agdefc | feabc bcdafe age eg\ngecdba ebdfg gcdef ecf cefadb fgac cf ecgafd cbfgead adgec | dfecg afcg bcfead ecadg\ngd cbfad fdagb cfbeag fabge efabdg aged bdgfec dgf gbfadec | acefgb eabfgc becagf bfgda\nebgc fedabcg fdbgce fdebg eg badgf ebcdf edg adcfeb cfgade | bgefd cbgefd bgefd abfdg\ndgbfc abecfg gcdab fcgdbe dfge cbdfea defbc fgc dabgefc gf | gf dbgecf bafgec cgf\ndegbac fda cdbag eafgbcd df fdbc agfdcb dabfg fbgea fcgade | fd bdceafg fdagbce df\ncedaf fgeabc egdbf gbaedcf aeg cgda dfaeg cfdbea fagdce ga | febadc gefad bfacde gae\ngea ebfgdc bcae cgafd abecfgd gbced ea gbdeaf dcgae gebcda | efgdab fcegdb cbgade acged\ncdabgef gb fceag fgb bfdgac gbcfa cbadfe dfcegb fbdca bgda | bg cbgfa dcfgeb afcgb\nfcbage adefc gceda bdegca cbeag dgeb efacdgb cfbgda adg dg | gad gabced gebd dg\necbdga gedbf dafeg faecbdg eacfg dbaf ad dbfcge gda dfbeag | ad gfbcde dgfea aecfg\nagfbde begfca bca baegc bc bcef ecdgbfa adegc bgaef acbfdg | fdbcag baecg cgdbaf bcdagf\nbeafc badfc daecfb fd fad fdec badefg cbdag fbecgad gecfab | dcfe cbgeaf gdcfabe agdbc\ncaedgbf fcgead ca gbadf abcd adcfbg fegbc dfaebg gfbac agc | fcgeda dbac afcgb dafebg\ngdfeb gdbafe bc ecb ebfagdc bgfce gfeca fdcbge aebdcf bcdg | cdfbeg gdbfe gefcb dbcafe\ngfbca gcdfe dbafgc cafgbe eacfbgd cdb agdb db cgdbf ecdbaf | adfcbe abdgfc cdb fcabed\nbcdaf fbed edbac cdaegf ed dbgaecf edc ebgac dbagfc fdbace | cbgae efdb gcdafe gbafedc\ncdfba cbdfae cfga bafdgc aedfgbc dbgef dag adgfb bdaegc ag | ebacgd adfgcb bdaefc gfac\ncaefd ce abfdc egcbdf cfe fgaced bdgfea gcae fadcbge eagfd | fcdae fgecad ec cbefgd\neafbd deb aefdg bd aecfbg bdcf abcfe gebcdaf agdbec bcaedf | dbcfae abfecd efabcd cbafe\nbdafeg efg gfcdae bagfd dfacgb ef dgfecba befa efbdg dbceg | fe gadbf aebfdg afeb\ncgbef ceb bfdgcae gedbac acgfbe be gceafd eacfg fcdgb fbea | abcedg dcgefa be fcegadb\ngacb gfbaedc fagdc baf gadcef bfcdea fgebd gfabd cfdgba ba | baf cadfg gbfad fab\ngafce df cbdfge gfd gdecb gecdf fdeb cadbeg agdbcf abgdcef | cgfea abgcde decgf fgcdbea\negdbf cbfgde aed befa gfdbae ea abcgd edfcga bcaegdf agdbe | bfae cagbfde cbgda gedcaf\neb dfbacge dbgae becafg abe gadfb cdega cedagb ecfgad debc | cfgeda fagedc afdbg fdcega\nefcba becagd gafcdbe eafdbg dagbcf agfbd gefd de bfaed deb | fabce bgaedc ceadbg bed\ncbaedf fdgebca gdbe dabce eag ge bacge bagcf decfga bgecda | defgabc bceagd aeg gbacf\ndgeabf aefgcdb ad bcfae bdacf dacg bgfdc ebfdgc gfdbac abd | dcga adgc decfbg bafce\nfgcba cbdfeag dagfb dcgbaf dcaegb ecbafg bdg bd fcbd faegd | bgdaec feadg cbdage dcgafb\nbdc dcfgeb ebgca bdea bdcga abfecg gdcaf bd aecdbfg aebgdc | bade bdecgf bdc cbadg\nbcdaeg facgbd caedfb aefdb dgfbe eba ae dcegfab fcea fbcad | cbafed baecdf ae ceabfd\nefcbg egd dg cabgef bfdceag fgcbde fdcea gdfb dgebca dfcge | fdgb gd fbgd deg\ncbgdfa ebgcfa abdge bdeca efcgbad cd fbedac abecf adc edcf | agebd gfabedc dabfegc abfce\nedg abdgce gcefb dcbge dgabfe gcdab de cdebfga cdae fdabcg | gbdafc agcdb dgfceab bafgdec\nacdb dgbfec eagfcdb dafbec cae ebdfc ca gfaed acdef gfebac | defac begdfc daegf fdeacb\ncgedf gfadce debgcf fedagcb aefbc bcdagf db ebfcd bfd begd | db cgfde dbefc gedcfb\nafcbegd dcfge edgbf bdg fabd dabfeg gaebdc abgecf gfeab db | debacg gfbaec fadbegc afcgbe\nfcbg cdegf ecdga eacdfb befdg dcf fc dfegba dbfgce agdfcbe | dcf adcge fbcg dgaefbc\nbcfea fcbead ecd cgeafb aebcgd bfed bcgedfa de cadfg fedac | de egadfbc debf bfagec\nefcdabg afecbd defba cabfd ebca cgdaf dfabeg bc efcdbg fbc | bgdefc afcgebd gdefcb efabgd\nedbaf agfbcde gbfcae ag dega aefcdb dfbega dfgbc afdgb bag | dagefb ga decbfa aecbgf\ncbdg aegbcfd badce dgaebf abdcfe gad cgeda gd fcage ceagbd | fdcaeb dbeca beafdc bdace\ndecb dagfe dcgbafe fecbda acfdb adfbcg agefbc fec ec faced | fcadeb cdagfb agbfce gcfdba\nacdbef dgca gbfae agecfdb ebdcg bda bgeda gedbfc ad bcadge | cgdbe cdag dcga efdcgab\ngc efbdg eadcf ebcafg adecgf gfdbaec gcf gcda dcgfe dcbaef | gc acedbf fcead gdca\nbfgce dabfg ecdf cebgfa dfegb ed deb fecbgda becgda cfbedg | cdgbefa ebd gafdb cdgefba\nce gecb ecd debaf ecdfb dcfega dagcbef fbgcd bdcgaf dcgfeb | dec dfbec agcfed bedfa\ncgbfd gb dcafg gadb gbfcea bcfdeag fcbde fbg gcbfad agdfec | dcfgab bfgdc dfaceg dfgac\nbgacef cdagf bgdcae gd dag dbagfc fecagbd fdbg cfead agbfc | gfcba adgcf facgb gd\nefdc adbgc gec acfgde feadg gbecaf fbdgae agdec daefbgc ce | ec cedf cge bdfagce\naecdbg cabfe acfgeb bcefda fgac fdgeb afdcbge bcg cebfg gc | gcbfae febcda facg baefcg\ndgbafce gfacdb gecb dcaefg gfaeb egf gebacf bdefa bgcaf eg | abfge fgabe fge deagfc\nceafdb dcbega afd gdbeaf fdgea fgeac gbade cbfadeg fd dfbg | adbcge gdcfeab afd fd\ndacegf ed dfcbg cfgea dcfge fcgdbae acgbef ced eagd abefcd | dfbeac fgcdb geda dbfgc\negbcdf ecbdga afegc aefdbgc dgeca dge dg dcfbae dgab cdbea | gcead eabdcf gdeac cfadbe\ngca fceagd fdgbc ga fecab fgcabed bgcaf cdbfge adbg acdfgb | agdb bfadcg bfgac gbfca\nacgdeb baefd fa gdfa bgdea bdcfe fdagebc fdgbea ecfgba fab | adbecg agcbed febagc feagcdb\nfedagc dcfge ef bgdcf gdceba egf fead edcag gfbaec fdgaebc | cgade aecfdg efg eadf\ndbagf gcdefab fc badfc cbaed gfadbe dgfc gfbcad gaebfc bcf | cfb cdbea bdagf fc\nbae be gcadeb dbge dgebacf eagcd geabc fbcga eagfdc edbafc | gcabf ecdfbag afbcg cbgfa\nbd gdbcf cbfegd cfbeag febdagc fbd fcgeb decb afgbed dfgac | cbefg eadcbfg cbegfad egdfcb\nfebacg dega cegfd cefda ae agebcfd abcdf eca defacg ecgfbd | badcf cae bdcefg acedf\ngeabcd gdbcfa gaedc cbeagf bdgeacf gdefc bdacg ae adbe cae | gcebad agfbdc gefbcad ea\nfa bfdacge adecgb eacf bdfgac gfdbe aegdc egacfd gadfe fga | gedfb egfbd efagd dagfbc\ngcdb dg beagdf feacg cebgdfa afbcd adcgf dbfcga ebfdac agd | gd acdfg dcbaf gacfe\naefgbd cgfdb gfdea eabfgc dcgfe cfe ceda gdcaef ce fdeabgc | bdcgf edgaf cbdfg egfbda\nfacegb cfdabeg bd cedgbf adcfeb cfabe cdb eadb cgdfa dfbca | dfbca eadb adecbgf bdc\nbacfeg agfcdeb acegf gfcade ecagbd fdbag afegd cdfe ed edg | dfce egd degaf dagfb\ndf gdfcea efbadg cegafbd eacfd fad cedbga dgaec dfcg fbcea | caedg dgafbe edgac df\nbfdac cdbgfa cefbgd bfag afgbdec cdgafe cbfdg acf ecbda fa | dgcfae af cabfd beadc\nbefgd dea ecab baefcd gfbcad ea bafcd dbcgefa afebd cadfeg | gfbadc eda cadgfb eda\ngf cgadb gebf becfdga gaefcd febac gcbaf cbfdea bfgeac fag | fg afcbg efbg afg\nba aebg gafdceb bca bdacg dagcf fcbdae gcbed cadebg bgcefd | dcagf gdabc afgcd edcfgb\nde dbec bfaecdg gdfeca fegcb edg dbgaf fceabg febcgd bgdef | afdbg adbfg debfgc bdgfa\nafbced adebfg efagdbc caebf afgec ecgb ega eg fgdac acegfb | aedgbf cbge egbfda badfgec\nfg gbfcdea eafbcd fdaeb cdage egf agdefb fdcbge efgda fgab | deacg cdage gedca adfeb\ngde gbdc dg fdgec dfaegb fedca bcgefd fbeacg gadecbf fcbeg | cgfabe edcgf fgeabdc cbefg\nbefcdg agbcef fcbdeag gdfae bdecf eab fcdeab ab efbad bcad | cfgeba befda aefgd degbcfa\nabcef dbfaegc aefcg dcgbae fbcg efgacb cg cdabfe gec dfeag | dgfae gdefa agcbde afbced\ndgf fcbega afdbeg fgabe dg efadg bged adfbceg agbcfd fedca | aefgb begd fceda debg\ncdgaeb ba befgdca defbc gdecaf bae gabc afgdeb gedac decab | fbecd bae gdecfa edcba\nebagfd dfg dcbaeg dgbceaf gf gacdf fcade gacbd gcfb fbagcd | adgfc acbgd edbagf degabc\ngba eagbcf gb gbacf dacgebf bceg gcafed acfeg acbfd adegfb | abfcdeg dbcfage faecg afebgc"
  # "926558 low"
  # "be cfbegad cbdgef fgaecd cgeb fdcge agebfd fecdb fabcd edb | fdgacbe cefdb cefbgd gcbe\nedbfga begcd cbg gc gcadebf fbgde acbgfd abcde gfcbed gfec | fcgedb cgb dgebacf gc\nfgaebd cg bdaec gdafb agbcfd gdcbef bgcad gfac gcb cdgabef | cg cg fdcagb cbg\nfbegcd cbd adcefb dageb afcb bc aefdc ecdab fgdeca fcdbega | efabcd cedba gadfec cb\naecbfdg fbg gf bafeg dbefa fcge gcbea fcaegb dgceab fcbdga | gecf egdcabf bgf bfgea\nfgeab ca afcebg bdacfeg cfaedg gcfdb baec bfadeg bafgc acf | gebdcfa ecba ca fadegcb\ndbcfg fgd bdegcaf fgec aegbdf ecdfab fbedc dacgb gdcebf gf | cefg dcbef fcge gbcadfe\nbdfegc cbegaf gecbf dfcage bdacg ed bedf ced adcbefg gebcd | ed bcgafe cdgba cbgef egadfb cdbfeg cegd fecab cgb gbdefca cg fgcdab egfdb bfceg | gbdfcae bgc cg cgb\ngcafb gcf dcaebfg ecagb gf abcdeg gaef cafbge fdbac fegbdc | fgae cfgab fg bagce"
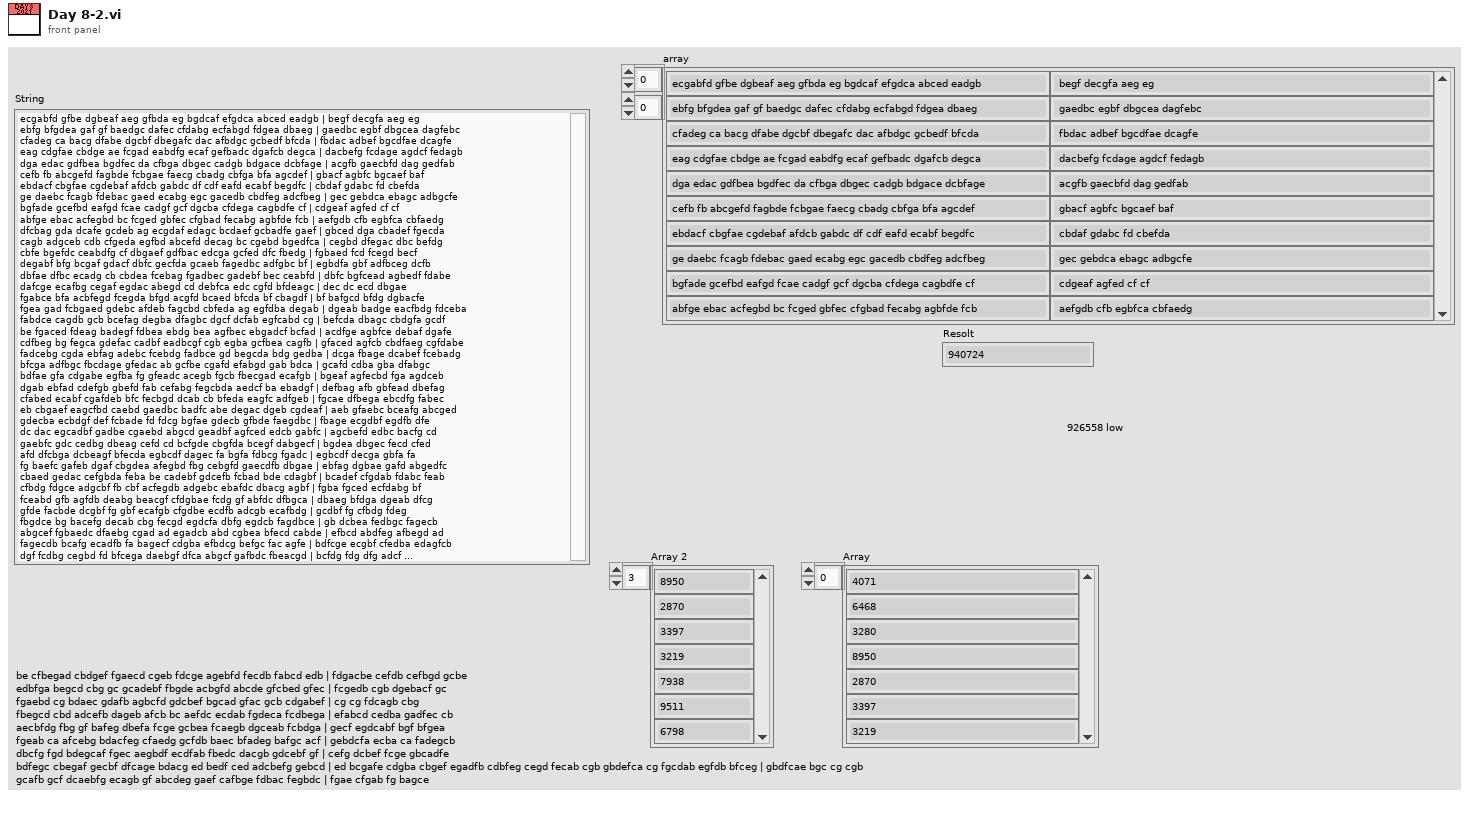
[diagram p1: front panel]
types:
  T1 = typedef "Day 8.lvlib/Digit.ctl" = cluster{"Number":u8, "Letters":string}
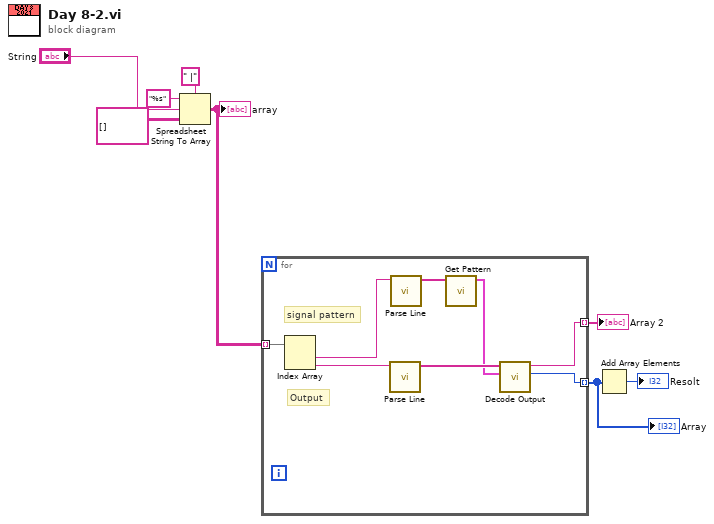
[diagram p0: block diagram]
diagram:
  n1 = Spreadsheet String To Array(delimiter (Tab)=" |", format string="%s", spreadsheet string="String", array type (2D Dbl)=string[][] []) -> (array=w1:string[][])
  "array" <- w1
  n2 = for {
    tunnel: [w16] -> w4 mode=indexing
    tunnel: [w15] -> w2 mode=indexing
    tunnel: w1 -> [w14] mode=indexing
    # "Output"
    # "signal pattern"
    n3 = Index Array(array=w14) -> (element #1=w13:string, element #2=w12:string)  [unwired: 2 in]
    n4 = call "Parse Line.vi"("format string"=w12) -> ("array type (2D Dbl)"=w11:string[])  [unwired: 10 in]
    n5 = call "Parse Line.vi"("format string"=w13) -> ("array type (2D Dbl)"=w10:string[])  [unwired: 10 in]
    n6 = call "Get Pattern.vi"("Signal Patern"=w10) -> ("appended array"=w9:T1[])  [unwired: 10 in]
    n7 = call "Decode Output.vi"("Map of numbers"=w9, "array type (2D Dbl)"=w11) -> ("Numeric"=w16:i32, "String"=w15:string)  [unwired: 8 in]
  }
  "Array" <- w4
  "Array 2" <- w2
  n8 = Add Array Elements(numeric array=w4) -> (sum=→"Resolt":i32)
